vi "Command Response.vi"(8 "error in (no error)":errorcluster, 10 "Message":refnum<class "Message Interface.lvclass">, 11 "WS Server in":refnum<class "WS Server.lvclass">) -> (0 "error out":errorcluster, 3 "WS Server out":refnum<class "WS Server.lvclass">)   [LabVIEW 2016, in "WebSocket Networking.lvlib" / "WS Server.lvclass"]
uses:
  <userlib>/Common Components/WebSocket Networking/WS Server/WS Server.lvclass
  C:/Program Files (x86)/National Instruments/LabVIEW 2016/user.lib/Composed Systems/Stream/Mediator/Classes/Websocket Server Actor/Websocket Server/Websocket Server.lvclass
  C:/Program Files (x86)/National Instruments/LabVIEW 2016/user.lib/Composed Systems/Stream/Mediator/Classes/Mediated Asynchronous Actor/Mediated Asynchronous Actor.lvclass
  <userlib>/Composed Systems/Stream/Mediator/Classes/Message Interface/Message Interface.lvclass
  <userlib>/Composed Systems/Stream/Mediator/Classes/Message Command Stop/Stop Msg.lvclass
  <userlib>/Composed Systems/Stream/Mediator/Classes/Message Interface/Message Interface.lvclass/Message Interface.ctl
  <userlib>/Composed Systems/Stream/Mediator/Classes/Message Transport Queue/Message Transport Queue.lvclass
  C:/Program Files (x86)/National Instruments/LabVIEW 2016/user.lib/Composed Systems/Stream/Mediator/Classes/Message Transport Interface/Message Transport Interface.lvclass
  <userlib>/Composed Systems/Stream/Mediator/Classes/Websocket Server Actor/Websocket Server/Websocket Server.lvclass
  <userlib>/Composed Systems/Stream/Mediator/Classes/Websocket Client Handler Actor/Websocket Client Handler Msgs/Write Msg/Write Msg.lvclass
  <userlib>/Composed Systems/Stream/Mediator/Classes/Mediated Asynchronous Actor/Mediated Asynchronous Actor.lvclass
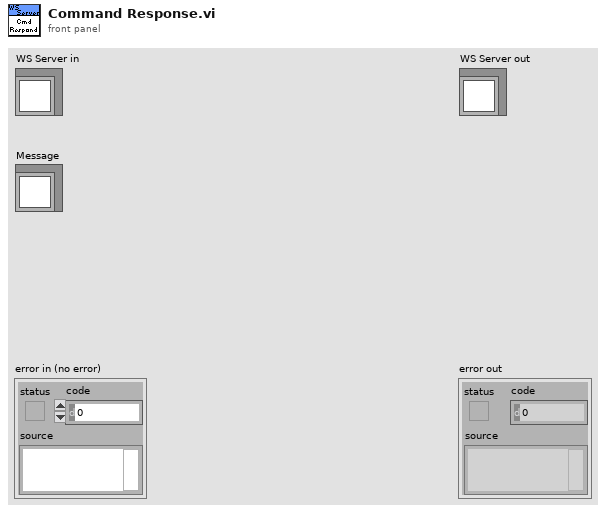
[diagram p1: front panel]
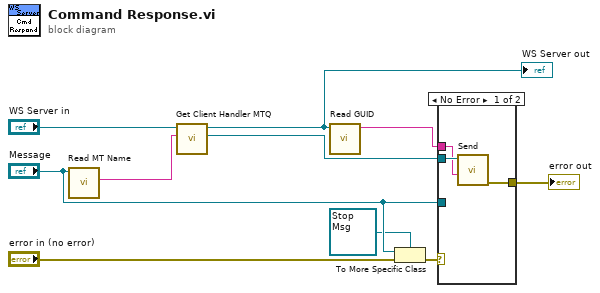
[diagram p0: block diagram]
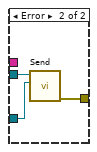
[diagram p2: hidden frame]
diagram:
  n1 = call <userlib>:"Read MT Name.vi"("Message Interface in"="Message") -> ("MT Name"=w9:string)  [unwired: 9 in, 1 out]
  n2 = call <userlib>:"Get Client Handler MTQ.vi"("GUID"=w9, "Websocket Server in"="WS Server in") -> ("Websocket Client Handler MTQ"=w8:refnum<class "Message Transport Queue.lvclass">, "Websocket Server out"=w2:refnum<class "WS Server.lvclass">)  [unwired: 6 in, 2 out]
  "WS Server out" <- w2
  n3 = call <userlib>:"Read GUID.vi"("Mediated Asynchronous Actor in"=w2) -> ("GUID"=w1:string)  [unwired: 10 in]
  n4 = To More Specific Class(target class=refnum<class "Stop Msg.lvclass"> refnum ("Stream Mediator.lvlib:Stop Msg.lvclass"), reference="Message", error in="error in (no error)") -> (error out=w4:errorcluster)  [unwired: 1 out]
  n5 = case shown="No Error" w4 {
    tunnel: w8 -> [w13 w16]
    tunnel: [w12 w15] -> w7
    tunnel: "Message" -> [_ w14]
    tunnel: w1 -> [w11 _]
    frame No Error {
      n6 = call <userlib>:"Send.vi"("Caller Actor Name"=w11, "Message Transport"=w13) -> ("error out"=w12:errorcluster)  [unwired: 9 in]
    }
    frame Error {
      n7 = call <userlib>:"Send.vi"("Message"=w14, "Message Transport Queue"=w16) -> ("error out"=w15:errorcluster)  [unwired: 9 in]
    }
  }
  "error out" <- w7
